vi "VolkAn(Walk Analyzer).vi"() -> ()   [LabVIEW 2017]
uses:
  <vilib>/LabVIEW Interface for Arduino/Type Defs/Board Type.ctl
  <vilib>/LabVIEW Interface for Arduino/Type Defs/Connection Type.ctl
  <vilib>/LabVIEW Interface for Arduino/LabVIEW Interface for Arduino.lvlib
panel:
  in  "Programı Durdurmak İçin Basınız!":bool
  in  "Bağlantı Noktasını Seçiniz!":refnum<visa-resource-name>
  out "Basınç Kuvveti Yoğunluk Grafiği":dbl[][](graph)
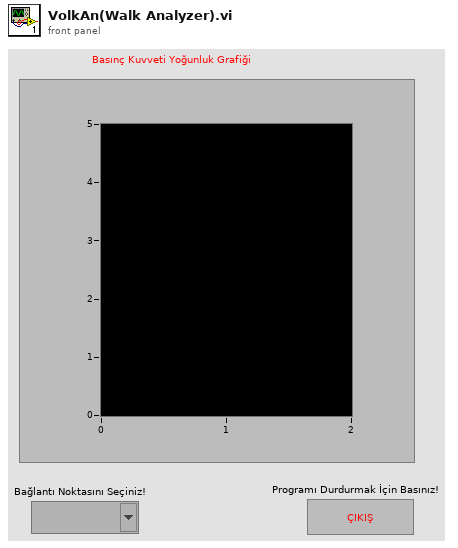
[diagram p1: front panel]
types:
  T1 = typedef "LabVIEW Interface for Arduino.lvlib/Connection Type.ctl" = enum8{"USB / Serial", "XBEE", "BlueSmirf (Bluetooth)"}
  T2 = typedef "LabVIEW Interface for Arduino.lvlib/Board Type.ctl" = enum16{"Uno", "Dimuelanove w/Atmega 328", "Mega 2560"}
  T3 = typedef "LabVIEW Interface for Arduino.lvlib/Arduino Resource.ctl" = cluster{"VISA resource":refnum<visa-resource-name>, "Board Type":T2, "Connection Type":enum8{"USB / Serial"}, "Bytes Per Packet (15)":u8}
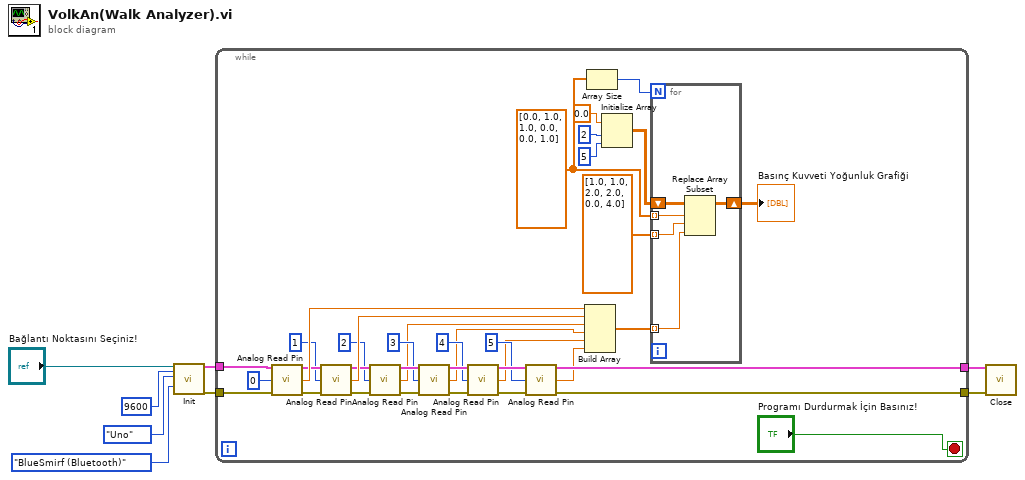
[diagram p0: block diagram]
diagram:
  n1 = call <vilib>:"Init.vi"("VISA resource"="Bağlantı Noktasını Seçiniz!", "Baud Rate (115200)"=u32 9600, "Board Type (Uno)"=Board_Type."Uno", "Connection Type (USB/Serial)"=Connection_Type."BlueSmirf (Bluetooth)") -> ("Arduino Resource"=w6:T3, "error out"=w4:errorcluster)  [unwired: 14 in]
  n2 = while {
    tunnel: w6 -> [w44]
    tunnel: [w25] -> w5
    tunnel: w4 -> [w43]
    tunnel: [w24] -> w3
    stop <- "Programı Durdurmak İçin Basınız!" stop-if-true
    w10 = dbl[] [0.0, 1.0, 1.0, 0.0, 0.0, 1.0] ("x")
    n3 = call <vilib>:"Analog Read Pin.vi"("Arduino Resource"=w44, "Analog Input Pin (0)"=u8 0, "error in"=w43) -> ("Arduino Resource"=w33:T3, "Voltage"=w35:dbl, "error out"=w32:errorcluster)  [unwired: 10 in]
    n4 = call <vilib>:"Analog Read Pin.vi"("Arduino Resource"=w33, "Analog Input Pin (0)"=u8 1, "error in"=w32) -> ("Arduino Resource"=w29:T3, "Voltage"=w30:dbl, "error out"=w23:errorcluster)  [unwired: 10 in]
    n5 = call <vilib>:"Analog Read Pin.vi"("Arduino Resource"=w29, "Analog Input Pin (0)"=u8 2, "error in"=w23) -> ("Arduino Resource"=w28:T3, "Voltage"=w15:dbl, "error out"=w22:errorcluster)  [unwired: 10 in]
    n6 = call <vilib>:"Analog Read Pin.vi"("Arduino Resource"=w28, "Analog Input Pin (0)"=u8 3, "error in"=w22) -> ("Arduino Resource"=w27:T3, "Voltage"=w14:dbl, "error out"=w21:errorcluster)  [unwired: 10 in]
    n7 = call <vilib>:"Analog Read Pin.vi"("Arduino Resource"=w27, "Analog Input Pin (0)"=u8 4, "error in"=w21) -> ("Arduino Resource"=w26:T3, "Voltage"=w13:dbl, "error out"=w20:errorcluster)  [unwired: 10 in]
    n8 = call <vilib>:"Analog Read Pin.vi"("Arduino Resource"=w26, "Analog Input Pin (0)"=u8 5, "error in"=w20) -> ("Arduino Resource"=w25:T3, "Voltage"=w12:dbl, "error out"=w24:errorcluster)  [unwired: 10 in]
    n9 = Build Array(w35, w30, w15, w14, w13, w12) -> (w34:dbl[])
    n10 = Array Size(array=w10) -> (size(s)=w39:i32)
    n11 = Initialize Array(0.0 ("element"), 2 ("dimension size"), 5 ("dimension size")) -> (w40:dbl[][])
    n12 = for {
      N: w39 -> [_]
      shift-right: [w46] -> w36
      shift-left: w40 -> [w49]
      tunnel: w10 -> [w48] mode=indexing
      tunnel: dbl[] [1.0, 1.0, 2.0, 2.0, 0.0, 4.0] ("y") -> [w47] mode=indexing
      tunnel: w34 -> [w45] mode=indexing
      n13 = Replace Array Subset(array=w49, new element=w45, index (row)=w48, index (col)=w47) -> (w46:dbl[][])
    }
    "Basınç Kuvveti Yoğunluk Grafiği" <- w36
  }
  n14 = call <vilib>:"Close.vi"("Arduino Resource"=w5, "error in"=w3) -> ()  [unwired: 13 in, 1 out]
